vi "DSF.Engine.Sequencer.Get Iteration.vi"(8 "error in (no error)":errorcluster, 11 "Sequencer Bundle in":refnum<class "Sequencer Bundle.lvclass">) -> (0 "error out":errorcluster, 2 "iteration":u64, 3 "Sequencer Bundle out":refnum<class "Sequencer Bundle.lvclass">)   [LabVIEW 2016, in "DSF.Engine.lvlib" / "Sequencer Bundle.lvclass"]
uses:
  Sequencer Bundle.lvclass
  Sequencer Bundle.lvclass/Sequencer Bundle.ctl
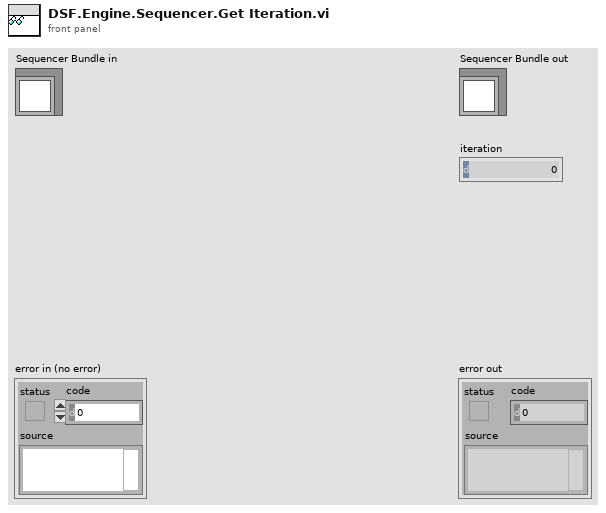
[diagram p1: front panel]
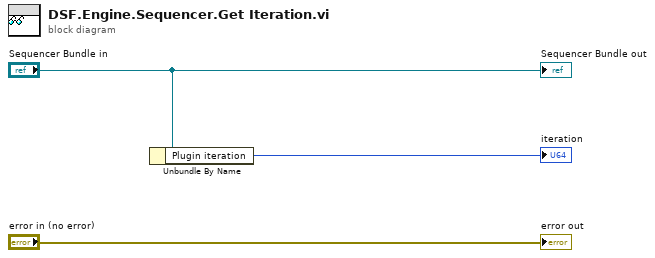
[diagram p0: block diagram]
diagram:
  n1 = Unbundle By Name("Sequencer Bundle in") -> ("Plugin iteration"=→"iteration":u64)
  "error out" <- "error in (no error)"
  "Sequencer Bundle out" <- "Sequencer Bundle in"
